vi "Calc - P1.vi"(11 "POIab":dbl) -> (3 "P1":dbl)   [LabVIEW 2018, in "Controller (Host).lvlib"]
uses:
  Controller (Host).lvlib
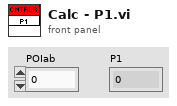
[diagram p1: front panel]
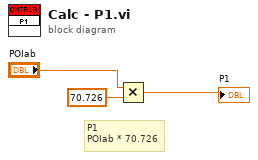
[diagram p0: block diagram]
diagram:
  # "P1\nPOIab * 70.726"
  n1 = Multiply(x="POIab", y=70.726) -> (x*y=→"P1":dbl)
